vi "CheckFPGAUse.vi"(0 "Exp_params":T4={"filename"="201612181913", "ExpFilePath"=path "C:/Documents and Settings/Bauerle/Mes documents/takada/HBT6/201612181913.h5", "File Ref list"=[16777217, 33554433, 16777216, 33554432], "sweep_dim"=[11, 61, 61], "sweep_list"=["suq", "ruq", "rlq", "slq", "sur", "rur", "rlr", "slr", "suc", "ruc", "rlc", "slc"], "readout_list"=["sud", "rud", "rld", "sld"], "Sweep instrument bools"=[[0, 0], [0, 0], [0, 0], [0, 0], [0, 0], [0, 0], [0, 0], [0, 0], [0, 0], [0, 0], [0, 0], [0, 0], [0, 0], [0, 0], [0, 0], [0, 0], [0, 0], [0, 0], [0, 0], [0, 0], [0, 0], [0, 0], [0, 0], [0, 0], [0, 0], [0, 0], [0, 0], [0, 0], [0, 0], [0, 0], [0, 0], [0, 0], [0, 0], [0, 0], [0, 0], [0, 0], [0, 0], [0, 0], [0, 0], [0, 0], [0, 0]], "Read out instrument bools"=[[1, 0]], "Experimental bool list"=[TRUE, TRUE], "Initial move"=[{"Name"="None", "kind"=100, "Value"=0.0}], "FPGA Ref"=refnum, "Inst_parameters"={"ConfigFilePath"=path "\\\\10.0.0.7\\takada2/DATA/HBT6/data/Configs/conf_20161218_fc_load.h5", "Inst_list"=["ADC", "AWG", "Freq", "Power", "sus", "rus", "rls", "sls", "suq", "suu", "sur", "suc", "sul", "ruq", "ruu", "rur", "ruc", "rul", "rlq", "rlu", "rlr", "rlc", "rll", "slq", "slu", "slr", "slc", "sll", "tu", "t", "tl", "fast_sequence", "4:7", "suc_load", "sur_load", "ruc_load", "rur_load", "rlc_load", "rlr_load", "slc_load", "slr_load", "load_time"], "fast_mode"=[1, 0], "Wait_times"=[1, 1, 1, 1], "Inst_array"=[{"Kind"=0, "Strings"=["ADC", "", "V", "sud;rud;rld;sld", "nA;nA;nA;nA", "100.0;100.0;100.0;100.0"], "uint64s"=[5, 4, 250000, 1, 100, 10106, 1000000, 1, 0, 1], "Doubles"=[1.0], "DAQmx take out list"=[]}, {"Kind"=7, "Strings"=["AWG", "10.0.0.4", "", "C:\\Documents and Settings\\Bauerle\\Mes documents\\Bautze\\FPGA-clean_works_1.13.6_batchtest\\Python\\AWG", "dummy", "SAWnstrig_v4.py"], "uint64s"=[2, 0, 0, 3, 0, 0, 0, 0, 0, 0, 0, 0, 0, 0], "Doubles"=[1200000000.0, 1.0, 0.0, 1.0, 0.0, 1.0, 0.0, 1.0, 0.0, 1.0, 0.0, 1.0, 0.0], "DAQmx take out list"=[]}, {"Kind"=6, "Strings"=["Freq", "0:19", "GHz"], "uint64s"=[1, 0, 0, 0, 2, 0, 0, 0], "Doubles"=[2.0, -30.0, 200.0, 100.0, 0.0, 6.000999927520752, 9.000000318337698e-06, 30.0, -145.0], "DAQmx take out list"=[]}, {"Kind"=6, "Strings"=["Power", "0:19", "GHz"], "uint64s"=[1, 0, 1, 0, 2, 0, 0, 1], "Doubles"=[2.0, -30.0, 200.0, 100.0, 0.0, 6.000999927520752, 9.000000318337698e-06, 30.0, -145.0], "DAQmx take out list"=[]}, {"Kind"=4, "Strings"=["sus", "10.0.0.2", "mV"], "uint64s"=[0, 1], "Doubles"=[1.0, -1.0, 1.0, -1.0, 1.0], "DAQmx take out list"=[]}, {"Kind"=4, "Strings"=["rus", "10.0.0.2", "mV"], "uint64s"=[0, 2], "Doubles"=[1.0, -1.0, 1.0, -1.0, 1.0], "DAQmx take out list"=[]}, {"Kind"=4, "Strings"=["rls", "10.0.0.2", "mV"], "uint64s"=[0, 3], "Doubles"=[1.0, -1.0, 1.0, -1.0, 1.0], "DAQmx take out list"=[]}, {"Kind"=4, "Strings"=["sls", "10.0.0.2", "mV"], "uint64s"=[0, 4], "Doubles"=[1.0, -1.0, 1.0, -1.0, 1.0], "DAQmx take out list"=[]}, {"Kind"=4, "Strings"=["suq", "10.0.0.2", "V"], "uint64s"=[0, 5], "Doubles"=[0.30000001192092896, -2.0, 1.0, -1.0, 1.0], "DAQmx take out list"=[]}, {"Kind"=4, "Strings"=["suu", "10.0.0.2", "V"], "uint64s"=[0, 6], "Doubles"=[0.30000001192092896, -2.0, 1.0, -1.0, 1.0], "DAQmx take out list"=[]}, {"Kind"=4, "Strings"=["sur", "10.0.0.2", "V"], "uint64s"=[0, 7], "Doubles"=[0.30000001192092896, -2.0, 1.0, -1.0, 1.0], "DAQmx take out list"=[]}, {"Kind"=4, "Strings"=["suc", "10.0.0.2", "V"], "uint64s"=[1, 0], "Doubles"=[0.30000001192092896, -2.0, 1.0, -1.0, 1.0], "DAQmx take out list"=[]}, {"Kind"=4, "Strings"=["sul", "10.0.0.2", "V"], "uint64s"=[1, 1], "Doubles"=[0.30000001192092896, -2.0, 1.0, -1.0, 1.0], "DAQmx take out list"=[]}, {"Kind"=4, "Strings"=["ruq", "10.0.0.2", "V"], "uint64s"=[1, 2], "Doubles"=[0.30000001192092896, -2.0, 1.0, -1.0, 1.0], "DAQmx take out list"=[]}, {"Kind"=4, "Strings"=["ruu", "10.0.0.2", "V"], "uint64s"=[1, 3], "Doubles"=[0.30000001192092896, -2.0, 1.0, -1.0, 1.0], "DAQmx take out list"=[]}, {"Kind"=4, "Strings"=["rur", "10.0.0.2", "V"], "uint64s"=[1, 5], "Doubles"=[0.30000001192092896, -2.0, 1.0, -1.0, 1.0], "DAQmx take out list"=[]}, {"Kind"=4, "Strings"=["ruc", "10.0.0.2", "V"], "uint64s"=[1, 6], "Doubles"=[0.30000001192092896, -2.0, 1.0, -1.0, 1.0], "DAQmx take out list"=[]}, {"Kind"=4, "Strings"=["rul", "10.0.0.2", "V"], "uint64s"=[1, 7], "Doubles"=[0.30000001192092896, -2.0, 1.0, -1.0, 1.0], "DAQmx take out list"=[]}, {"Kind"=4, "Strings"=["rlq", "10.0.0.2", "V"], "uint64s"=[2, 0], "Doubles"=[0.30000001192092896, -2.0, 1.0, -1.0, 1.0], "DAQmx take out list"=[]}, {"Kind"=4, "Strings"=["rlu", "10.0.0.2", "V"], "uint64s"=[2, 1], "Doubles"=[0.30000001192092896, -2.0, 1.0, -1.0, 1.0], "DAQmx take out list"=[]}, {"Kind"=4, "Strings"=["rlr", "10.0.0.2", "V"], "uint64s"=[2, 2], "Doubles"=[0.30000001192092896, -2.0, 1.0, -1.0, 1.0], "DAQmx take out list"=[]}, {"Kind"=4, "Strings"=["rlc", "10.0.0.2", "V"], "uint64s"=[2, 3], "Doubles"=[0.30000001192092896, -2.0, 1.0, -1.0, 1.0], "DAQmx take out list"=[]}, {"Kind"=4, "Strings"=["rll", "10.0.0.2", "V"], "uint64s"=[2, 4], "Doubles"=[0.30000001192092896, -2.0, 1.0, -1.0, 1.0], "DAQmx take out list"=[]}, {"Kind"=4, "Strings"=["slq", "10.0.0.2", "V"], "uint64s"=[2, 5], "Doubles"=[0.30000001192092896, -2.0, 1.0, -1.0, 1.0], "DAQmx take out list"=[]}, {"Kind"=4, "Strings"=["slu", "10.0.0.2", "V"], "uint64s"=[2, 6], "Doubles"=[0.30000001192092896, -2.0, 1.0, -1.0, 1.0], "DAQmx take out list"=[]}, {"Kind"=4, "Strings"=["slr", "10.0.0.2", "V"], "uint64s"=[2, 7], "Doubles"=[0.30000001192092896, -2.0, 1.0, -1.0, 1.0], "DAQmx take out list"=[]}, {"Kind"=4, "Strings"=["slc", "10.0.0.2", "V"], "uint64s"=[3, 0], "Doubles"=[0.30000001192092896, -2.0, 1.0, -1.0, 1.0], "DAQmx take out list"=[]}, {"Kind"=4, "Strings"=["sll", "10.0.0.2", "V"], "uint64s"=[3, 1], "Doubles"=[0.30000001192092896, -2.0, 1.0, -1.0, 1.0], "DAQmx take out list"=[]}, {"Kind"=4, "Strings"=["tu", "10.0.0.2", "V"], "uint64s"=[3, 2], "Doubles"=[0.30000001192092896, -2.0, 1.0, -1.0, 1.0], "DAQmx take out list"=[]}, {"Kind"=4, "Strings"=["t", "10.0.0.2", "V"], "uint64s"=[3, 3], "Doubles"=[0.30000001192092896, -2.0, 1.0, -1.0, 1.0], "DAQmx take out list"=[]}, {"Kind"=4, "Strings"=["tl", "10.0.0.2", "V"], "uint64s"=[3, 4], "Doubles"=[0.30000001192092896, -2.0, 1.0, -1.0, 1.0], "DAQmx take out list"=[]}, {"Kind"=9, "Strings"=["fast_sequence", "10.0.0.2", "V"], "uint64s"=[6661, 300, 100, 0, 7, 8, 5, 13, 14, 10, 18, 19, 16, 23, 24, 21, 26, 27, 28, 39, 0], "Doubles"=[1.0, -1.0, -1.0, -1.0], "DAQmx take out list"=[]}, {"Kind"=4, "Strings"=["4:7", "10.0.0.2", "V"], "uint64s"=[4, 7], "Doubles"=[0.30000001192092896, -2.0, 1.0, -1.0, 1.0], "DAQmx take out list"=[]}, {"Kind"=10, "Strings"=["suc_load", "10.0.0.2", "V"], "uint64s"=[4, 0], "Doubles"=[0.5, -0.5], "DAQmx take out list"=[]}, {"Kind"=10, "Strings"=["sur_load", "10.0.0.2", "V"], "uint64s"=[5, 0], "Doubles"=[0.5, -0.5], "DAQmx take out list"=[]}, {"Kind"=10, "Strings"=["ruc_load", "10.0.0.2", "V"], "uint64s"=[6, 0], "Doubles"=[0.5, -0.5], "DAQmx take out list"=[]}, {"Kind"=10, "Strings"=["rur_load", "10.0.0.2", "V"], "uint64s"=[7, 0], "Doubles"=[0.5, -0.5], "DAQmx take out list"=[]}, {"Kind"=10, "Strings"=["rlc_load", "10.0.0.2", "V"], "uint64s"=[8, 0], "Doubles"=[0.5, -0.5], "DAQmx take out list"=[]}, {"Kind"=10, "Strings"=["rlr_load", "10.0.0.2", "V"], "uint64s"=[9, 0], "Doubles"=[0.5, -0.5], "DAQmx take out list"=[]}, {"Kind"=10, "Strings"=["slc_load", "10.0.0.2", "V"], "uint64s"=[10, 0], "Doubles"=[0.5, -0.5], "DAQmx take out list"=[]}, {"Kind"=10, "Strings"=["slr_load", "10.0.0.2", "V"], "uint64s"=[11, 0], "Doubles"=[0.5, -0.5], "DAQmx take out list"=[]}, {"Kind"=10, "Strings"=["load_time", "10.0.0.2", "ms"], "uint64s"=[12, 0], "Doubles"=[1000.0, -0.009999999776482582], "DAQmx take out list"=[]}]}} {"File Ref list" format="%.0x"}) -> (1 "use FPGA":bool, 2 "IP address":string, 3 "DAC lock-in":T1, 4 "FPGA ADC":T1)   [LabVIEW 2013]
uses:
  <vilib>/addons/h5labview2/base/hid_t.ctl
  fpga-bitfile-ref.ctl
panel:
  out "start read vals":bool=TRUE
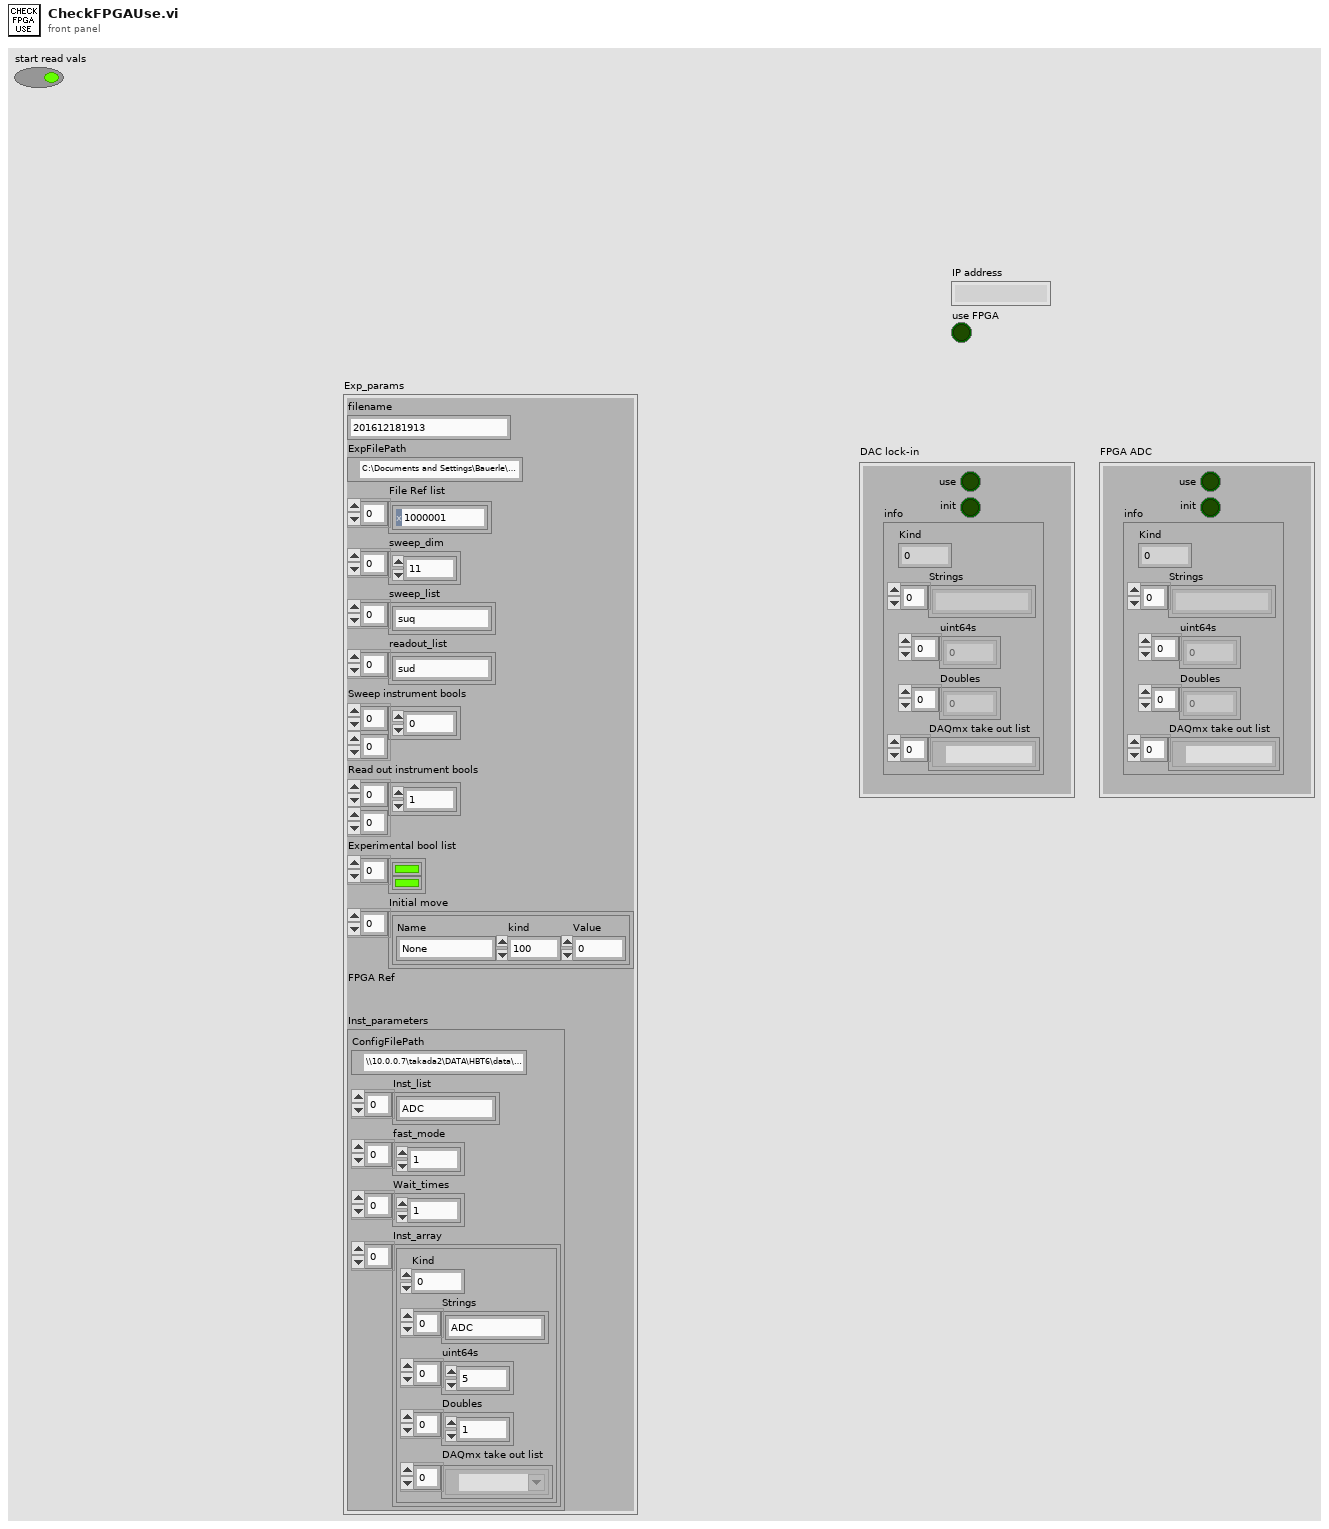
[diagram p1: front panel]
types:
  T1 = cluster{"use":bool, "init":bool, "info":cluster{"Kind":u16, "Strings":string[], "uint64s":u64[], "Doubles":dbl[], "DAQmx take out list":refnum<k21>[]}}
  T2 = typedef "hid_t.ctl" = i32
  T3 = typedef "fpga-bitfile-ref.ctl" = refnum<k20>
  T4 = cluster{"filename":string, "ExpFilePath":path, "File Ref list":T2[], "sweep_dim":u64[], "sweep_list":string[], "readout_list":string[], "Sweep instrument bools":u64[][], "Read out instrument bools":u64[][], "Experimental bool list":bool[], "Initial move":cluster{"Name":string, "kind":u64, "Value":dbl}[], "FPGA Ref":T3, "Inst_parameters":cluster{"ConfigFilePath":path, "Inst_list":string[], "fast_mode":u8[], "Wait_times":u64[], "Inst_array":cluster{"Kind":u16, "Strings":string[], "uint64s":u64[], "Doubles":dbl[], "DAQmx take out list":refnum<k21>[]}[]}}
  T5 = cluster{"Kind":u16, "Strings":string[], "uint64s":u64[], "Doubles":dbl[], "DAQmx take out list":refnum<k21>[]}[]
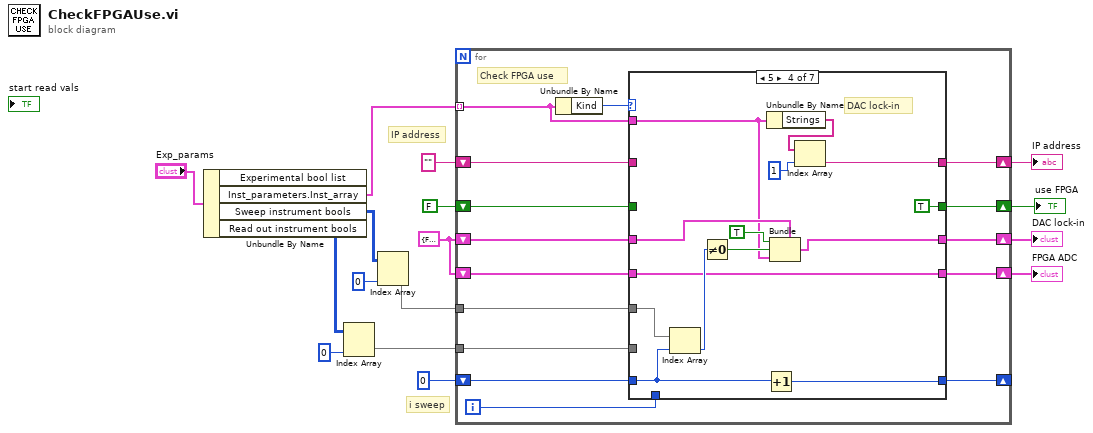
[diagram p0: block diagram]
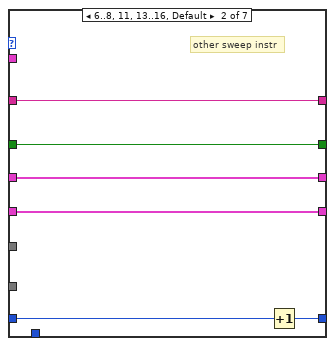
[diagram p3: hidden frame]
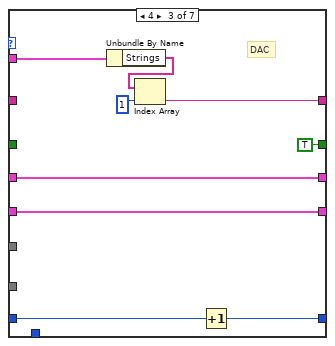
[diagram p4: hidden frame]
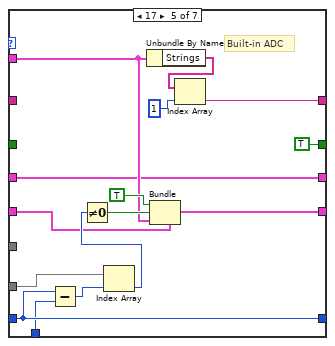
[diagram p5: hidden frame]
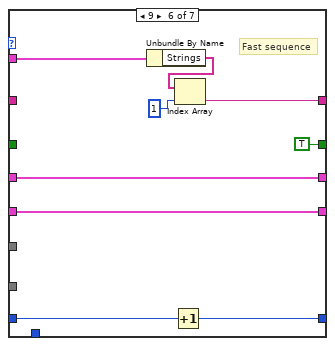
[diagram p6: hidden frame]
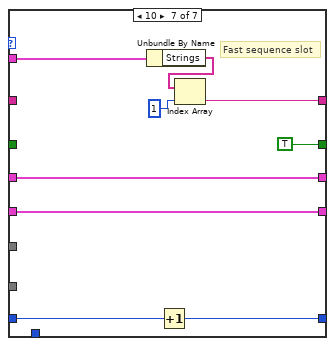
[diagram p7: hidden frame]
diagram:
  w7 = T1 {"use"=FALSE, "init"=FALSE, "info"={"Kind"=0, "Strings"=[], "uint64s"=[], "Doubles"=[], "DAQmx take out list"=[]}} ("DAC lock-in")
  # "IP address"
  # "i sweep"
  n1 = Unbundle By Name("Exp_params") -> ("Inst_parameters.Inst_array"=w15:T5, "Sweep instrument bools"=w14:u64[][], "Read out instrument bools"=w1:u64[][])  [unwired: 1 out]
  n2 = Index Array(array=w1, index (col)=0) -> (element=w2:u64[])  [unwired: 1 in]
  n3 = Index Array(array=w14, index (col)=0) -> (element=w13:u64[])  [unwired: 1 in]
  n4 = for {
    tunnel: w15 -> [w28] mode=indexing
    shift-right: [w30] -> w4
    shift-left: FALSE -> [w31]
    shift-right: [w27] -> w5
    shift-left: "" -> [w29]
    shift-right: [w25] -> w8
    shift-left: w7 -> [w26]
    tunnel: w13 -> [w20]
    shift-right: [w23] -> _
    shift-left: 0 -> [w19]
    shift-right: [w21] -> w6
    shift-left: w7 -> [w22]
    tunnel: w2 -> [w17]
    i -> [w18]
    # "Check FPGA use"
    n5 = Unbundle By Name(w28) -> ("Kind"=w24:u16)
    n6 = case shown="5" w24 {
      tunnel: w31 -> [w36 w40 _ _ _ _ _]
      tunnel: [w36 w40 TRUE TRUE TRUE TRUE TRUE] -> w30
      tunnel: w29 -> [w35 w41 _ _ _ _ _]
      tunnel: w28 -> [_ _ w50 w55 w74 w88 w97]
      tunnel: [w35 w41 w43 w63 w78 w85 w94] -> w27
      tunnel: w26 -> [w34 w42 w47 w58 w72 w84 w93]
      tunnel: [w34 w42 w47 w54 w72 w84 w93] -> w25
      tunnel: w20 -> [_ _ _ w61 _ _ _]
      tunnel: w19 -> [w33 w38 w46 w60 w69 w83 w92]
      tunnel: [w33 w39 w45 w62 w69 w81 w91] -> w23
      tunnel: [w32 w37 w44 w53 w71 w82 w90] -> w21
      tunnel: w22 -> [w32 w37 w44 w53 w70 w82 w90]
      tunnel: w18 -> [_ _ _ _ w68 _ _]
      tunnel: w17 -> [_ _ _ _ w66 _ _]
      frame 0..3, 12 {
        # "other readout instr"
      }
      frame 6..8, 11, 13..16, Default {
        # "other sweep instr"
        n7 = Increment(x=w38) -> (x+1=w39:i32)
      }
      frame 4 {
        # "DAC"
        n8 = Unbundle By Name(w50) -> ("Strings"=w49:string[])
        n9 = Index Array(array=w49, index=1) -> (element=w43:string)
        n10 = Increment(x=w46) -> (x+1=w45:i32)
      }
      frame 5 {
        # "DAC lock-in"
        n11 = Index Array(array=w61, index=w60) -> (element=w56:u64)
        n12 = Not Equal To 0?(x=w56) -> (x != 0?=w57:bool)
        n13 = Increment(x=w60) -> (x+1=w62:i32)
        n14 = Unbundle By Name(w55) -> ("Strings"=w65:string[])
        n15 = Bundle(cluster=w58, "use"=TRUE, "init"=w57, "info"=w55) -> (w54:T1)
        n16 = Index Array(array=w65, index=1) -> (element=w63:string)
      }
      frame 17 {
        # "Built-in ADC"
        n17 = Subtract(x=w69, y=w68) -> (x-y=w67:i32)
        n18 = Index Array(array=w66, index=w67) -> (element=w75:u64)
        n19 = Not Equal To 0?(x=w75) -> (x != 0?=w76:bool)
        n20 = Unbundle By Name(w74) -> ("Strings"=w80:string[])
        n21 = Bundle(cluster=w70, "use"=TRUE, "init"=w76, "info"=w74) -> (w71:T1)
        n22 = Index Array(array=w80, index=1) -> (element=w78:string)
      }
      frame 9 {
        # "Fast sequence"
        n23 = Unbundle By Name(w88) -> ("Strings"=w87:string[])
        n24 = Increment(x=w83) -> (x+1=w81:i32)
        n25 = Index Array(array=w87, index=1) -> (element=w85:string)
      }
      frame 10 {
        # "Fast sequence slot"
        n26 = Unbundle By Name(w97) -> ("Strings"=w96:string[])
        n27 = Increment(x=w92) -> (x+1=w91:i32)
        n28 = Index Array(array=w96, index=1) -> (element=w94:string)
      }
    }
  }
  "FPGA ADC" <- w6
  "DAC lock-in" <- w8
  "IP address" <- w5
  "use FPGA" <- w4
